vi "PacketGen_v2.vi"(0 "Hex Array":string[](array[string]), 5 "AOL_Globals":T2={"Imaging Protocol"=enum."AOL Z-Stack", "Number of POI"=0, "Number of Miniscans"=0, "Number of Trials"=0, "Number of Cycles "=0, "# Averaged Frames"=0, "Laser power (%)"=0, "Pockels (V)"=0.0, "Acquisition Length (sec)"=0.0, "Fill time (us)"=0.0, "POI Dwell time (us)"=0.0, "Miniscan Dwell time per pixel (us)"=0.0, "PMT 1"=0.0, "PMT 2"=0.0, "Back Apperture (mA)"=0.0, "Frame Size"=0, "Center Frequency"=0.0, "Field of View (norm)"=0.0, "DwellTime (us)"=0.0, "Wavelength (nm)"=0.0, "Zoom"=0.0, "AOL Z"=0.0, "AOL Mode"=enum."Raster", "GridXY"=0.0, "GridZ"=0.0, "TriggerPeriod (sec)"=0.0, "Number of Pixels in Miniscan"=0, "Experiment folder path"=path "", "X centre"=0.0, "Y centre"=0.0, "Angle (degrees)"=0.0, "Plane Mode"=0, "Threshold"=[], "Regenerate Chirps"=FALSE, "Rectangle ROI length (pixels)"=0, "Rectangle ROI height (pixels)"=0, "AOD fill"=4900, "StartupDelay"=0, "Samples Wait after Trigger"=5080, "Slip Cycle"=600000, "Add Cycle"=TRUE, "Functional Mode"=enum."Point", "Z Start"=0.0, "Z Stop"=0.0, "# Planes"=0} {"Plane Mode" items=["XY Plane", "XZ Plane", "YZ Plane", "arbitraryplane"]; "Frame Size" items=["100X100"=100, "128X128"=128, "200X200"=200, "256X256"=256, "512X512"=512, "1024x1024"=1024, "2048x2048"=2048]; "Back Apperture (mA)" format="%#.6g"; "Pockels (V)" format="%#.6g"; "PMT 2" format="%#.6g"; "PMT 1" format="%#.6g"; "Angle (degrees)" format="%#.6g"; "POI Dwell time (us)" format="%#.6g"}, 9 "Ny":i32, 11 "Nx":i32, 14 "Imaging Protocol":T1) -> (4 "HexPackets":string[](array[string]), 10 "Interrupted":bool, 13 "Repeat":i32, 15 "error out":errorcluster)   [LabVIEW 2017]
uses:
  Typedefs/Controls/AOL_Globals.ctl
  Typedefs/Imaging Protocols enum.ctl
  Typedefs/Frame Size.ctl
  Typedefs/AOL modes.ctl
  Typedefs/Plane Mode.ctl
  Typedefs/Functional Mode.ctl
  Global Variables/General Globals.vi
panel:
  out "Objective":i8=20
  in  "Protocol to save packets on":T1=enum."Functional Acquisition"
  in  "error in (no error)":errorcluster
  in  "Save Packets":bool
  out "Total Packets":i32
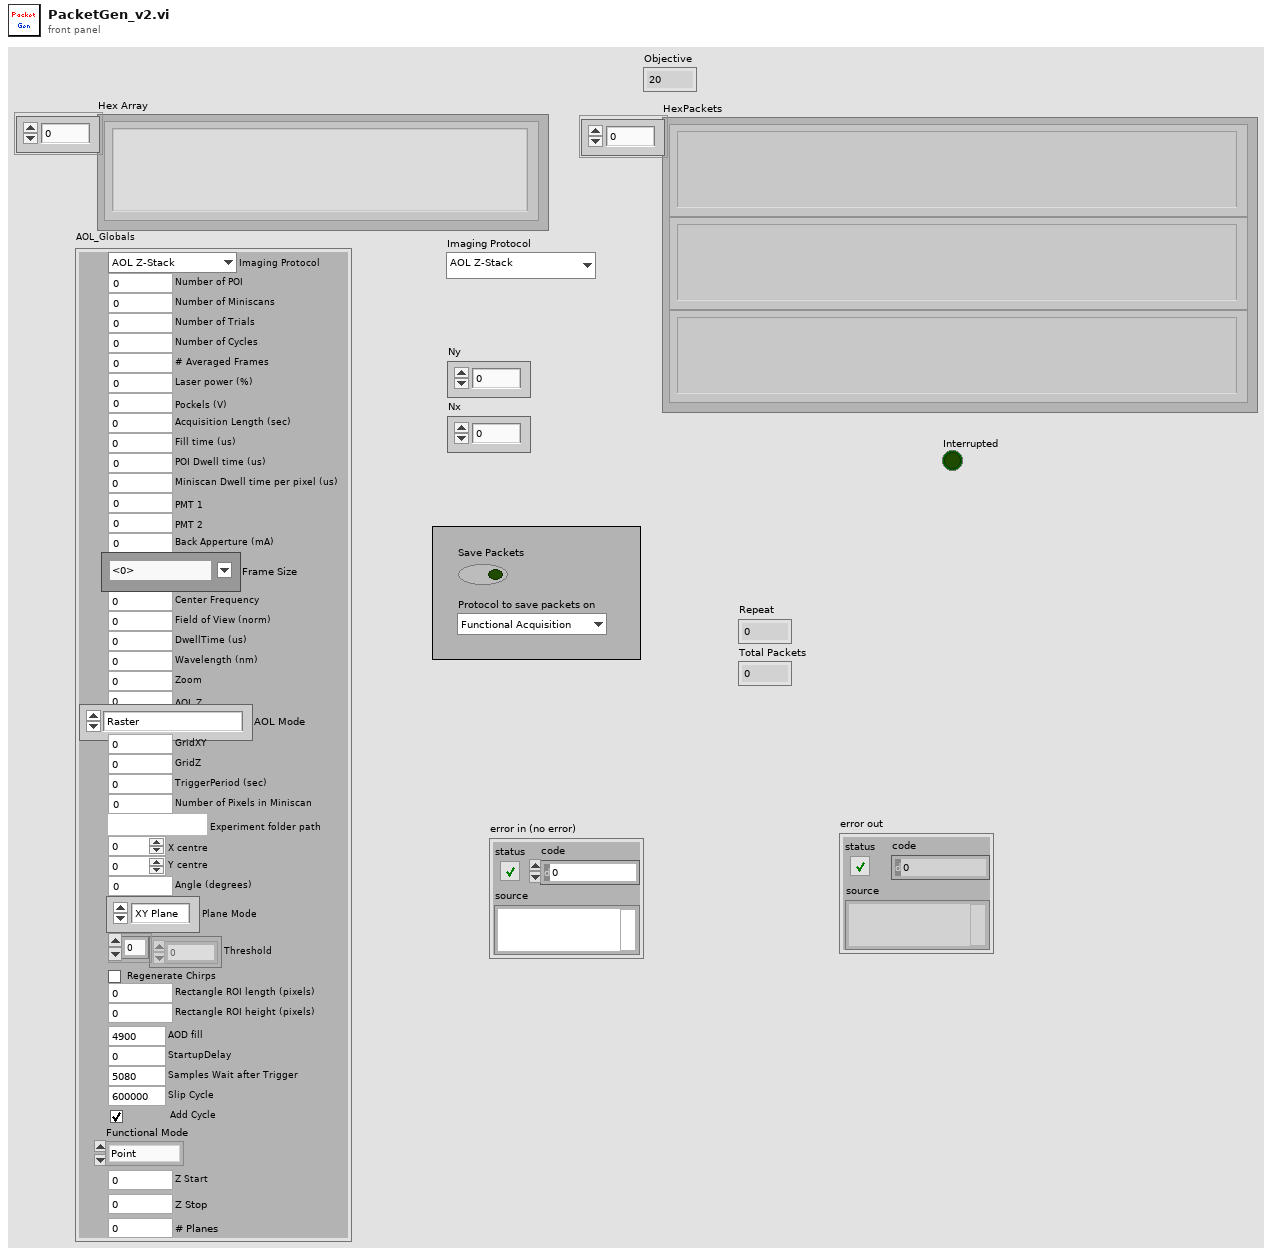
[diagram p1: front panel]
types:
  T1 = typedef "Imaging Protocols enum.ctl" = enum16{"AOL Z-Stack", "Motor Z Stack", "Functional Acquisition", "Single Plane Acquisition", "Volume Acquisition", "Live Imaging", "Live Plane Imaging", "Live Volume Imaging"}
  T2 = typedef "AOL_Globals.ctl" = cluster{"Imaging Protocol":T1, "Number of POI":u16, "Number of Miniscans":u16, "Number of Trials":u16, "Number of Cycles ":u64, "# Averaged Frames":u16, "Laser power (%)":u8, "Pockels (V)":dbl, "Acquisition Length (sec)":dbl, "Fill time (us)":dbl, "POI Dwell time (us)":dbl, "Miniscan Dwell time per pixel (us)":dbl, "PMT 1":dbl, "PMT 2":dbl, "Back Apperture (mA)":dbl, "Frame Size":T3, "Center Frequency":dbl, "Field of View (norm)":dbl, "DwellTime (us)":dbl, "Wavelength (nm)":dbl, "Zoom":dbl, "AOL Z":dbl, "AOL Mode":T4, "GridXY":dbl, "GridZ":dbl, "TriggerPeriod (sec)":dbl, "Number of Pixels in Miniscan":u16, "Experiment folder path":path, "X centre":dbl, "Y centre":dbl, "Angle (degrees)":dbl, "Plane Mode":T5, "Threshold":u16[], "Regenerate Chirps":bool, "Rectangle ROI length (pixels)":u16, "Rectangle ROI height (pixels)":u16, "AOD fill":u16, "StartupDelay":i32, "Samples Wait after Trigger":u16, "Slip Cycle":u32, "Add Cycle":bool, "Functional Mode":T6, "Z Start":dbl, "Z Stop":dbl, "# Planes":i32}
  T3 = typedef "Frame Size.ctl" = u16
  T4 = typedef "AOL modes.ctl" = enum16{"Raster", "Structural", "Pointing", "Mini Scan", "Alignment"}
  T5 = typedef "Plane Mode.ctl" = u16
  T6 = typedef "Functional Mode.ctl" = enum16{"Point", "Line", "Patch", "Plane", "Volume"}
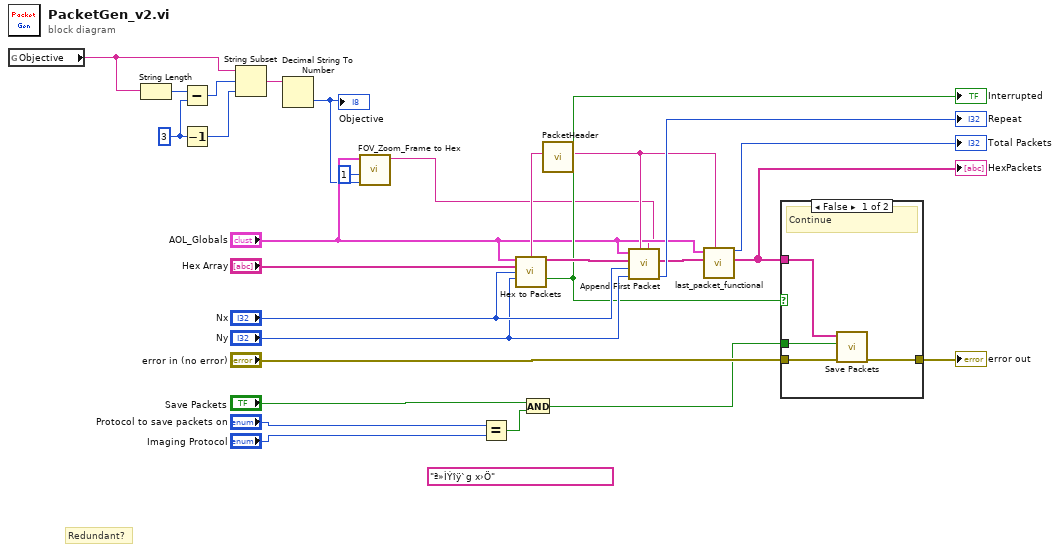
[diagram p0: block diagram]
diagram:
  w8 = 3
  (unwired) "ª»ÌÝîÿ`g x›Ö" ("PacketHeader")
  # "Redundant?"
  n1 = global read "General Globals.vi" "Objective"() -> (w3:string)
  n2 = String Length(string=w3) -> (length=w7:i32)
  n3 = Subtract(x=w7, y=w8) -> (x-y=w9:i32)
  n4 = Decrement(x=w8) -> (x-1=w10:i32)
  n5 = String Subset(string=w3, offset (0)=w9, length (rest)=w10) -> (substring=w6:string)
  n6 = Decimal String To Number(string=w6) -> (number=w2:i32)  [unwired: 2 in, 1 out]
  "Objective" <- w2
  n7 = call "FOV_Zoom_Frame to Hex.vi"("Objective"=w2, "Z pixel Size"=i8 1, "AOL_Globals"="AOL_Globals") -> ("FOV-Zoom-FrameSize Hex"=w4:string)  [unwired: 8 in]
  n8 = Equal?(x="Protocol to save packets on", y="Imaging Protocol") -> (x = y?=w14:bool)
  n9 = And(x="Save Packets", y=w14) -> (x .and. y?=w12:bool)
  n10 = call "PacketHeader.vi"() -> ("PacketHeader"=w11:string)  [unwired: 11 in]
  n11 = call "Hex to Packets.vi"("AOL_Globals"="AOL_Globals", "MAC Address"=w11, "Hex Array"="Hex Array", "Nx"="Nx", "Ny"="Ny") -> ("Packets"=w25:string[], "Interrupted"=w17:bool)  [unwired: 9 in]
  "Interrupted" <- w17
  n12 = call "Append First Packet.vi"("FOV-Zoom-FrameSize Hex"=w4, "MAC Address"=w11, "Ny"="Ny", "Nx"="Nx", "Packets"=w25, "AOL_Globals"="AOL_Globals") -> ("Repeat"=→"Repeat":i32, "HexPackets"=w22:string[])  [unwired: 3 in, 1 out]
  n13 = call "last_packet_functional.vi"("MAC Address"=w11, "Packets"=w22, "AOL_Globals"="AOL_Globals") -> ("HexPackets"=w21:string[], "Total Packets"=→"Total Packets":i32)  [unwired: 6 in, 1 out]
  "HexPackets" <- w21
  n14 = case shown="False" w17 {
    tunnel: w12 -> [w31 _]
    tunnel: "error in (no error)" -> [w30 w32]
    tunnel: [w29 w32] -> w23
    tunnel: w21 -> [w28 _]
    frame False {
      # "Continue"
      n15 = call "Save Packets.vi"("error in (no error)"=w30, "Save Packets"=w31, "Packets in"=w28) -> ("error out"=w29:errorcluster)  [unwired: 8 in]
    }
    frame True {
      # "Interrupted"
    }
  }
  "error out" <- w23
